vi "Ocean Optics 2000 4000 Process Spectrum.vi"() -> ()   [LabVIEW 2013]
doc: "Demonstrates measuring and processing the spectra and display in Absorbance, Transmission and Irradiance mode.\n\n<b>Note:</b>\nRefer to Spectrum Processing.vi for more details regarding the modes."
uses:
  <instrlib>/Ocean Optics 2000 4000/Ocean Optics 2000 4000.lvlib
panel:
  in  "Stop":bool
  out "Waveform":T1(graph)
  in  "Color Temperature (2850 K)":dbl=2850.0
  in  "Spectral Mode (0:Absorbance)":u16(ring) items=["Absorbance", "Transmission", "Irradiance"]
  in  "Read Reference":bool
  in  "Read Dark":bool
  in  "VISA resource name":refnum<visa-resource-name>
  # "(c) 2009 -213 National Instruments.  ALL RIGHTS RESERVED."
  # "To run this Example, select the spectral processing mode. Then run the VI. To read the dark spectrum, click Read Dark. Then click Read Reference to read Reference Spectrum. The processed spectrum will display on the graph. Press Stop when done."
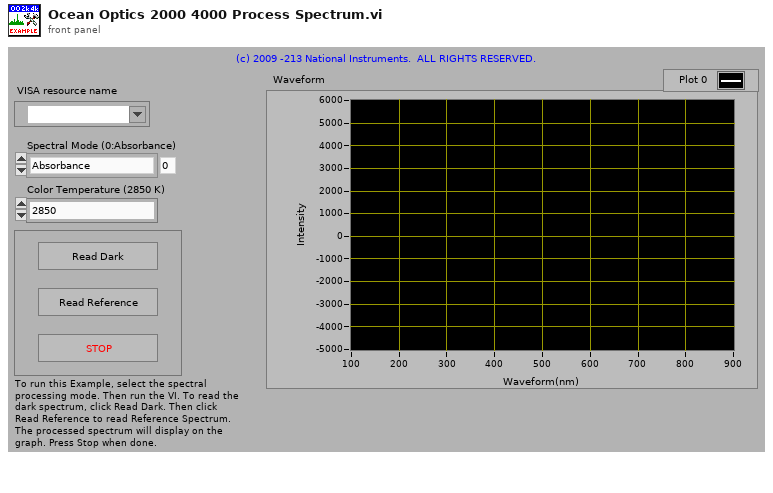
[diagram p1: front panel]
types:
  T1 = cluster{"Wavelength (nm)":dbl[], "Processed Spectrum":dbl[]}
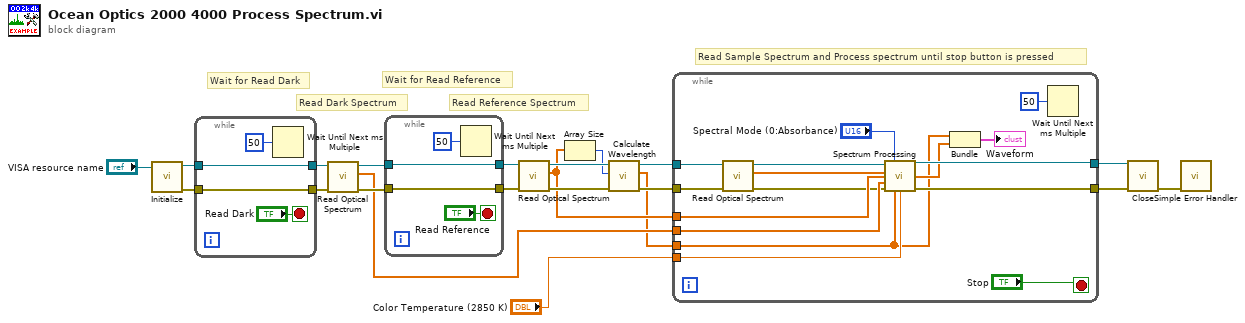
[diagram p0: block diagram]
diagram:
  # "Read Sample Spectrum and Process spectrum until stop button is pressed"
  # "Read Reference Spectrum"
  # "Read Dark Spectrum"
  # "Wait for Read Reference"
  # "Wait for Read Dark"
  n1 = call <instrlib>:"Initialize.vi"("VISA resource name"="VISA resource name") -> ("error out"=w19:errorcluster, "VISA resource name out"=w20:refnum<visa-resource-name>)  [unwired: 9 in]
  n2 = while {
    tunnel: [w24] -> w18
    tunnel: w20 -> [w24]
    tunnel: [w23] -> w17
    tunnel: w19 -> [w23]
    stop <- "Read Dark" stop-if-true
    n3 = Wait Until Next ms Multiple(millisecond multiple=u32 50) -> ()  [unwired: 1 out]
  }
  n4 = call <instrlib>:"Read Optical Spectrum.vi"("error in (no error)"=w17, "VISA resource name"=w18) -> ("error out"=w15:errorcluster, "Spectrum by Pixels"=w12:dbl[], "VISA resource name out"=w16:refnum<visa-resource-name>)  [unwired: 6 in, 1 out]
  n5 = while {
    tunnel: [w28] -> w13
    tunnel: w16 -> [w28]
    tunnel: [w27] -> w14
    tunnel: w15 -> [w27]
    stop <- "Read Reference" stop-if-true
    n6 = Wait Until Next ms Multiple(millisecond multiple=u32 50) -> ()  [unwired: 1 out]
  }
  n7 = call <instrlib>:"Read Optical Spectrum.vi"("error in (no error)"=w14, "VISA resource name"=w13) -> ("error out"=w10:errorcluster, "Spectrum by Pixels"=w9:dbl[], "VISA resource name out"=w11:refnum<visa-resource-name>)  [unwired: 6 in, 1 out]
  n8 = Array Size(array=w9) -> (size(s)=w8:i32)
  n9 = call <instrlib>:"Calculate Wavelength.vi"("error in (no error)"=w10, "Number of Pixels (3648)"=w8, "VISA resource name"=w11) -> ("error out"=w6:errorcluster, "Wavelength (nm)"=w5:dbl[], "VISA resource name out"=w7:refnum<visa-resource-name>)  [unwired: 6 in]
  n10 = while {
    tunnel: w12 -> [w45]
    tunnel: w9 -> [w44]
    tunnel: w7 -> [w42]
    tunnel: w6 -> [w43]
    tunnel: w5 -> [w33]
    tunnel: "Color Temperature (2850 K)" -> [w38]
    tunnel: [w37] -> w3
    tunnel: [w36] -> w2
    stop <- "Stop" stop-if-true
    n11 = call <instrlib>:"Read Optical Spectrum.vi"("error in (no error)"=w43, "VISA resource name"=w42) -> ("error out"=w40:errorcluster, "Spectrum by Pixels"=w39:dbl[], "VISA resource name out"=w41:refnum<visa-resource-name>)  [unwired: 6 in, 1 out]
    n12 = call <instrlib>:"Spectrum Processing.vi"("VISA resource name"=w41, "Spectral Mode (0:Absorbance)"="Spectral Mode (0:Absorbance)", "Sample Spectrum"=w39, "Reference Spectrum"=w44, "Dark Spectrum"=w45, "error in (no error)"=w40, "Wavelength (nm)"=w33, "Color Temperature (2850 K)"=w38) -> ("VISA resource name out"=w37:refnum<visa-resource-name>, "Processed Spectrum"=w34:dbl[], "error out"=w36:errorcluster)  [unwired: 5 in]
    n13 = Bundle("Wavelength (nm)"=w33, "Processed Spectrum"=w34) -> (→"Waveform":T1)  [unwired: 1 in]
    n14 = Wait Until Next ms Multiple(millisecond multiple=u32 50) -> ()  [unwired: 1 out]
  }
  n15 = call <instrlib>:"Close.vi"("error in (no error)"=w2, "VISA resource name"=w3) -> ("error out"=w1:errorcluster)  [unwired: 9 in]
  n16 = call <vilib>:"Simple Error Handler.vi"("error in (no error)"=w1) -> ()  [unwired: 4 in, 5 out]
